vi "AllOrFirstNot_comparison.vi"() -> ()   [LabVIEW 2013]
panel:
  out "first not time":u32
  out "or all time":u32
  out "first not":bool
  out "logical OR":bool
  out "ch array":dbl[][](array[numeric])
  in  "square array size":i32
  in  "ch col":i32
  in  "ch row":i32
  out "Array":dbl[][](array[numeric])
  # "Initialization:"
  # "Conclusions: With 1000 x 1000 array of doubles, comparing the logical or of all takes a fixed 5 ms. If the change is early, first not is faster; however, first not is slower for no change,\nor a change at the end. Therefore, there is no justification to coding the double first not loop."
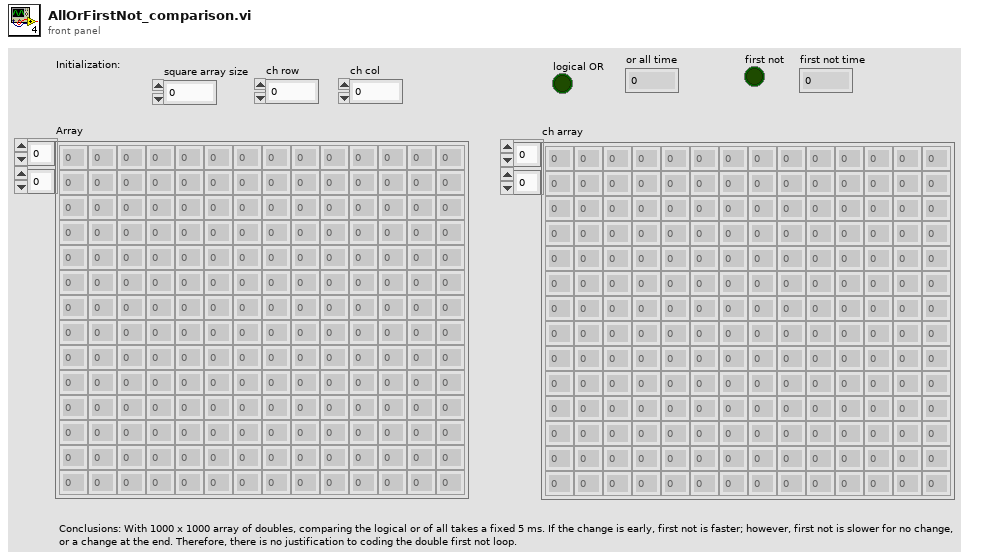
[diagram p1: front panel]
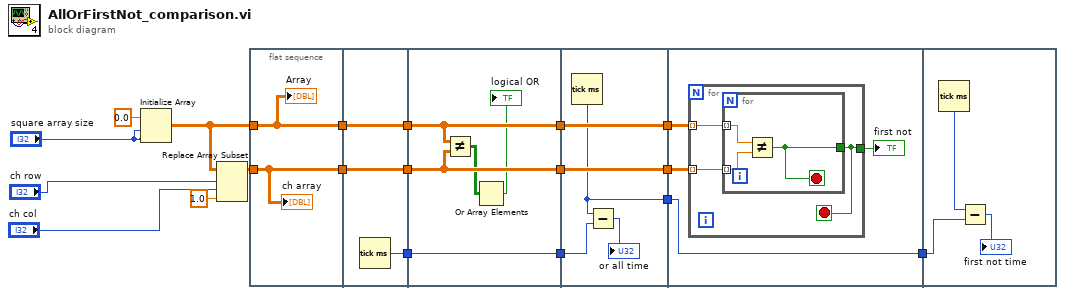
[diagram p0: block diagram]
diagram:
  n1 = Initialize Array(0.0 ("element"), "square array size", "square array size") -> (w17:dbl[][])
  n2 = Replace Array Subset(array=w17, new element=1.0 ("new element/subarray"), index (row)="ch row", index (col)="ch col") -> (w16:dbl[][])
  n3 = flat-sequence {
    tunnel: w17 -> [w21]
    tunnel: w16 -> [w20]
    tunnel: [w21] -> w12
    tunnel: [w20] -> w11
    tunnel: w12 -> [w24]
    tunnel: w11 -> [w23]
    tunnel: [w24] -> w10
    tunnel: [w23] -> w9
    tunnel: [w22] -> w1
    tunnel: w10 -> [w29]
    tunnel: w9 -> [w28]
    tunnel: [w29] -> w8
    tunnel: [w28] -> w7
    tunnel: [w25] -> w2
    tunnel: w1 -> [w25]
    tunnel: w8 -> [w34]
    tunnel: w7 -> [w33]
    tunnel: [w34] -> w6
    tunnel: [w33] -> w5
    tunnel: [w31] -> w3
    tunnel: w2 -> [w32]
    tunnel: w6 -> [w38]
    tunnel: w5 -> [w37]
    tunnel: [w35] -> w4
    tunnel: w3 -> [w35]
    tunnel: w4 -> [w46]
    frame #0 {
      "Array" <- w21
      "ch array" <- w20
    }
    frame #1 {
      n4 = Tick Count (ms)() -> (millisecond timer value=w22:u32)
    }
    frame #2 {
      n5 = Not Equal?(x=w29, y=w28) -> (x != y?=w27:bool[][])
      n6 = Or Array Elements(Boolean array=w27) -> (logical OR=→"logical OR":bool)
    }
    frame #3 {
      n7 = Tick Count (ms)() -> (millisecond timer value=w31:u32)
      n8 = Subtract(x=w31, y=w32) -> (x-y=→"or all time":u32)
    }
    frame #4 {
      n9 = for {
        tunnel: w38 -> [w41] mode=indexing
        tunnel: w37 -> [w40] mode=indexing
        tunnel: [w39] -> w36
        stop <- w39 stop-if-true
        n10 = for {
          tunnel: w41 -> [w44] mode=indexing
          tunnel: w40 -> [w43] mode=indexing
          tunnel: [w42] -> w39
          stop <- w42 stop-if-true
          n11 = Not Equal?(x=w44, y=w43) -> (x != y?=w42:bool)
        }
      }
      "first not" <- w36
    }
    frame #5 {
      n12 = Tick Count (ms)() -> (millisecond timer value=w45:u32)
      n13 = Subtract(x=w45, y=w46) -> (x-y=→"first not time":u32)
    }
  }
